vi "Update UI.vi"(8 "error in (no error)":errorcluster, 11 "Network Test in":refnum<class "Network Test.lvclass">) -> (0 "error out":errorcluster, 3 "Network Test out":refnum<class "Network Test.lvclass">)   [LabVIEW 2017, in "Network Test.lvlib" / "Network Test.lvclass"]
uses:
  Network Test.lvclass
  <vilib>/Utility/miscctls.llb/LVRowAndColumnTypeDef.ctl
  Network Test.lvclass/Network Test.ctl
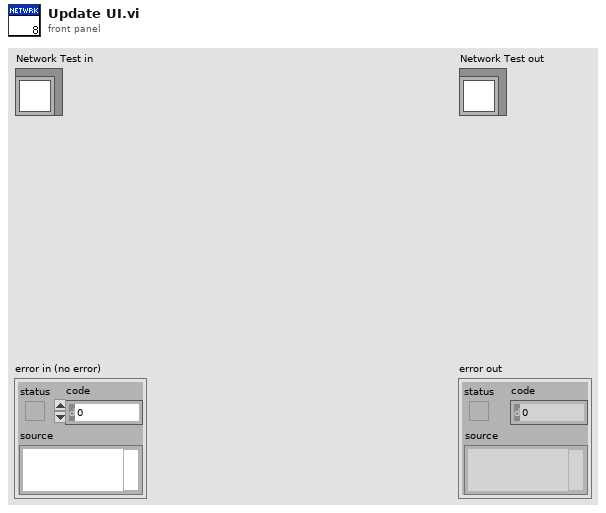
[diagram p1: front panel]
types:
  T1 = typedef "LVRowAndColumnTypeDef.ctl" = cluster{"Row":i32, "Column":i32}
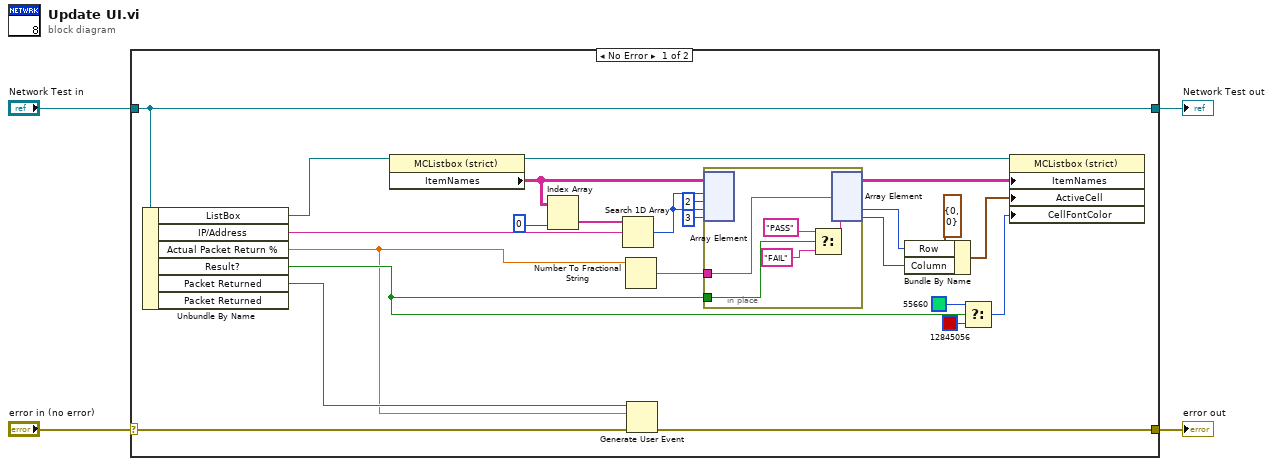
[diagram p0: block diagram]
diagram:
  n1 = case shown="No Error" "error in (no error)" {
    selector: "error in (no error)" -> [w10 w35]
    tunnel: [w9 w35] -> w3
    tunnel: [w28 w34] -> w1
    tunnel: "Network Test in" -> [w28 w34]
    frame No Error {
      n2 = Unbundle By Name(w28) -> ("ListBox"=w27:refnum<vi>, "IP/Address"=w24:string, "Actual Packet Return %"=w5:dbl, "Result?"=w15:bool, "Packet Returned"=w8:refnum<user-event>)  [unwired: 1 out]
      n3 = property class="MCListbox (strict)"(reference=w27) -> (reference out=w18:refnum<vi>, "ItemNames"=w23:string[][])  [unwired: 1 in, 1 out]
      n4 = Index Array(array=w23, index (col)=0 ("disabled index (col)")) -> (element=w25:string[])  [unwired: 1 in]
      n5 = Search 1D Array(1D array=w25, element=w24) -> (index of element=w21:i32)  [unwired: 1 in]
      n6 = Number To Fractional String(number=w5) -> (F-format string=w20:string)  [unwired: 3 in]
      n7 = Generate User Event(user event=w8, event data cluster=w5, error in=w10) -> (error out=w9:errorcluster)  [unwired: 1 in, 1 out]
      n8 = in-place {
        in-place-border: w15 -> [w33]
        in-place-border: w20 -> [w29]
        n9 = in-place-array #1(w23, w21, 2, w21, 3) -> ()  [unwired: 2 out]
        n10 = Select(t="PASS", s=w33, f="FAIL") -> (s? t:f=w30:string)
        n11 = in-place-array #1(w29, w30) -> (w6:string[][], w17:i32, w16:i32)  [unwired: 2 out]
      }
      n12 = Bundle By Name(cluster=T1 {"Row"=0, "Column"=0} ("Active Cell:Active Cell"), "Row"=w17, "Column"=w16) -> (w7:T1)
      n13 = Select(t=u32 55660 ("Color Box"), s=w15, f=u32 12845056 ("Color Box")) -> (s? t:f=w12:u32)
      n14 = property class="MCListbox (strict)"(reference=w18, "ItemNames"=w6, "ActiveCell"=w7, "CellFontColor"=w12) -> ()  [unwired: 1 in, 2 out]
    }
    frame Error {
    }
  }
  "error out" <- w3
  "Network Test out" <- w1
